vi "Fit VI window to Caller Center.vi"(4 "error in (no error)":errorcluster, 6 "Background VI Ref (Callee's Caller)":refnum<vi>, 7 "VI Ref (calling VI)":refnum<vi>) -> (0 "error out":errorcluster, 3 "VI Ref out":refnum<vi>)   [LabVIEW 2017]
doc: "Resizes and centres the window of VI Ref (calling VI) inside the window of the VI that called it."
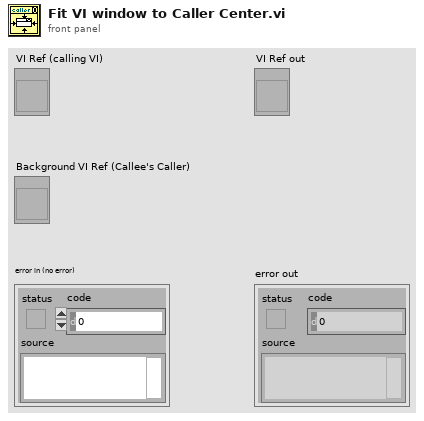
[diagram p1: front panel]
types:
  T1 = typedef "LVRectTypeDef.ctl" = cluster{"Left":i16, "Top":i16, "Right":i16, "Bottom":i16}
  T2 = cluster{"left":i16, "top":i16, "right":i16, "bottom":i16}
  T3 = typedef "LVAllMonitorsDisplayTypeDef.ctl" = cluster{"Bounds":cluster{"Left":i16, "Top":i16, "Right":i16, "Bottom":i16}, "Depth":i16}[]
  T4 = cluster{"Left":i16, "Top":i16, "Right":i16, "Bottom":i16}
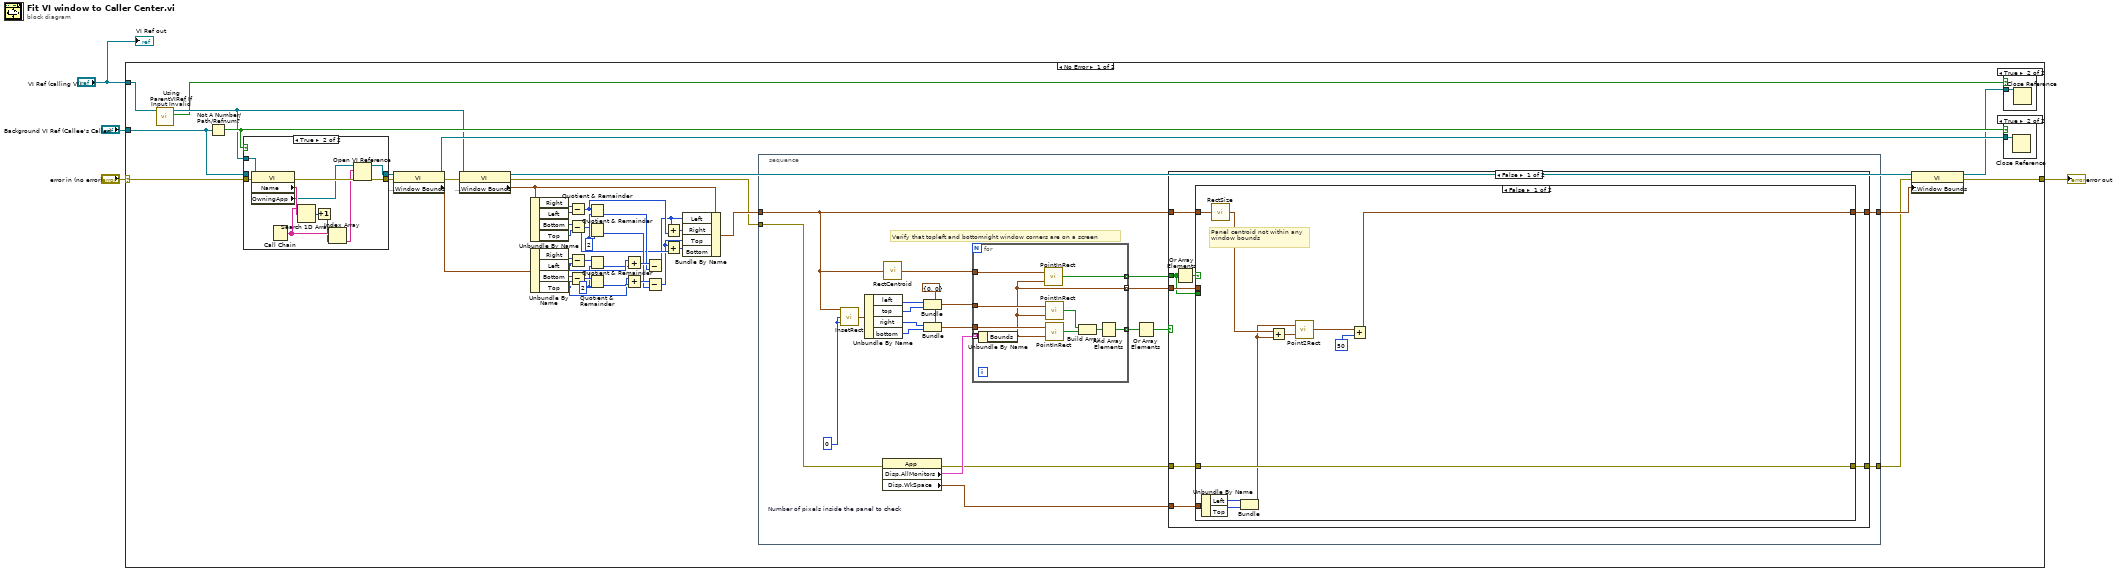
[diagram p0: block diagram]
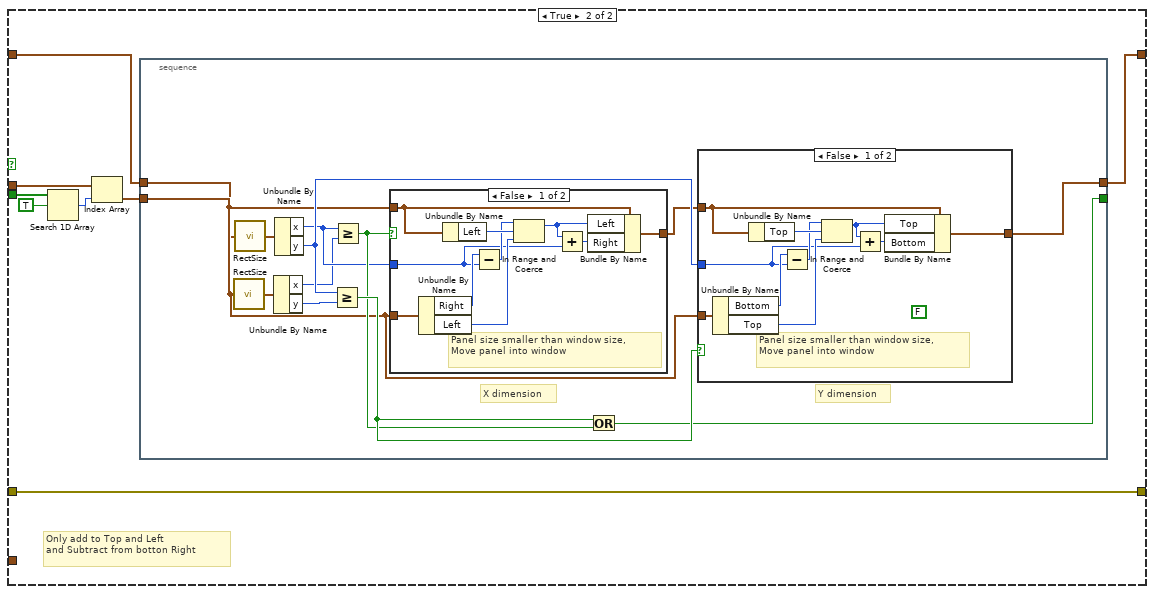
[diagram p2: hidden frame]
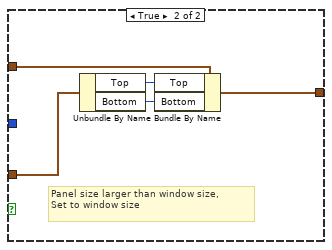
[diagram p3: hidden frame]
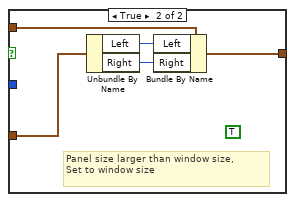
[diagram p4: hidden frame]
diagram:
  n1 = case shown="No Error" "error in (no error)" {
    selector: "error in (no error)" -> [w23 w166]
    tunnel: [w47 w166] -> w4
    tunnel: "Background VI Ref (Callee's Caller)" -> [w19 _]
    tunnel: "VI Ref (calling VI)" -> [w20 _]
    frame No Error {
      w40 = i16 2 ("y")
      w24 = i16 2 ("y")
      n2 = call "Using ParentVIRef If Input Invalid.vi"("VI Ref (calling VI)"=w20) -> ("Using Parent Ref(Need to Destroy)"=w7:bool, "VI Ref"=w15:refnum<vi>)  [unwired: 5 in]
      n3 = Not A Number/Path/Refnum?(number/path/refnum=w19) -> (NaN/Path/Refnum?=w21:bool)
      n4 = case shown="True" w21 {
        tunnel: w19 -> [w154 _]
        tunnel: [w154 w160] -> w18
        tunnel: w15 -> [_ w165]
        tunnel: w23 -> [w153 w164]
        tunnel: [w153 w161] -> w22
        frame False {
        }
        frame True {
          n5 = property class="VI"(reference=w165, error in=w164) -> (error out=w162:errorcluster, "Name"=w163:string, "OwningApp"=w157:refnum<vi>)  [unwired: 1 out]
          n6 = Call Chain() -> (call chain=w159:string[])
          n7 = Search 1D Array(1D array=w159, element=w163) -> (index of element=w156:i32)  [unwired: 1 in]
          n8 = Increment(x=w156) -> (x+1=w155:i32)
          n9 = Index Array(array=w159, index=w155) -> (element=w158:string)
          n10 = Open VI Reference(application reference (local)=w157, vi path=w158, error in (no error)=w162) -> (vi reference=w160:refnum<vi>, error out=w161:errorcluster)  [unwired: 3 in]
        }
      }
      n11 = property class="VI"(reference=w18, error in=w22) -> (reference out=w17:refnum<vi>, error out=w41:errorcluster, "Front Panel Window:Window Bounds"=w46:T1)
      n12 = property class="VI"(reference=w15, error in=w41) -> (reference out=w27:refnum<vi>, error out=w6:errorcluster, "Front Panel Window:Window Bounds"=w10:T1)
      n13 = Unbundle By Name(w10) -> ("Right"=w36:i16, "Left"=w37:i16, "Bottom"=w38:i16, "Top"=w39:i16)
      n14 = Unbundle By Name(w46) -> ("Right"=w45:i16, "Left"=w35:i16, "Bottom"=w44:i16, "Top"=w32:i16)
      n15 = Subtract(x=w36, y=w37) -> (x-y=w26:i16)
      n16 = Subtract(x=w38, y=w39) -> (x-y=w25:i16)
      n17 = Subtract(x=w45, y=w35) -> (x-y=w43:i16)
      n18 = Subtract(x=w44, y=w32) -> (x-y=w42:i16)
      n19 = Quotient & Remainder(x=w26, y=w40) -> (floor(x/y)=w30:i16)  [unwired: 1 out]
      n20 = Quotient & Remainder(x=w25, y=w40) -> (floor(x/y)=w28:i16)  [unwired: 1 out]
      n21 = Quotient & Remainder(x=w43, y=w24) -> (floor(x/y)=w34:i16)  [unwired: 1 out]
      n22 = Quotient & Remainder(x=w42, y=w24) -> (floor(x/y)=w33:i16)  [unwired: 1 out]
      n23 = Add(x=w35, y=w34) -> (x+y=w31:i16)
      n24 = Add(x=w32, y=w33) -> (x+y=w29:i16)
      n25 = Subtract(x=w31, y=w30) -> (x-y=w13:i16)
      n26 = Subtract(x=w29, y=w28) -> (x-y=w12:i16)
      n27 = Add(x=w13, y=w26) -> (x+y=w11:i16)
      n28 = Add(x=w12, y=w25) -> (x+y=w14:i16)
      n29 = Bundle By Name(cluster=w10, "Left"=w13, "Right"=w11, "Top"=w12, "Bottom"=w14) -> (w9:T1)
      n30 = stacked-sequence {
        tunnel: [w58] -> w5
        tunnel: [w49] -> w8
        tunnel: w6 -> [w51]
        tunnel: w9 -> [w65]
        frame #0 {
          w60 = i16 0  # Number of pixels inside the panel to check
          w64 = cluster{"x":i16, "y":i16} {"x"=0, "y"=0} ("point")
          # "Verify that topleft and bottomright window corners are on a screen"
          n31 = call <vilib>:"InsetRect.vi"("dv"=w60, "dh"=w60, "rect"=w65) -> ("inset rect"=w54:T2)
          n32 = Unbundle By Name(w54) -> ("left"=w52:i16, "top"=w53:i16, "right"=w61:i16, "bottom"=w62:i16)
          n33 = property class="App"(error in=w51) -> (error out=w48:errorcluster, "Disp.AllMonitors"=w50:T3, "Disp.WkSpace"=w59:T1)  [unwired: 1 in, 1 out]
          n34 = call <vilib>:"RectCentroid.vi"("rect"=w65) -> ("point"=w66:cluster{"x":i16, "y":i16})
          n35 = Bundle(cluster=w64, "x"=w52, "y"=w53) -> (w55:cluster{"x":i16, "y":i16})
          n36 = Bundle(cluster=w64, "x"=w61, "y"=w62) -> (w63:cluster{"x":i16, "y":i16})
          n37 = for {
            tunnel: w50 -> [w150] mode=indexing
            tunnel: w55 -> [w149]
            tunnel: [w145] -> w56 mode=indexing
            tunnel: w63 -> [w144]
            tunnel: w66 -> [w143]
            tunnel: [w142] -> w67 mode=indexing
            tunnel: [w141] -> w68 mode=indexing
            n38 = Unbundle By Name(w150) -> ("Bounds"=w141:T4)
            n39 = call <vilib>:"PointInRect.vi"("rect"=w141, "point"=w143) -> ("pt in rect"=w142:bool)
            n40 = call <vilib>:"PointInRect.vi"("rect"=w141, "point"=w149) -> ("pt in rect"=w148:bool)
            n41 = call <vilib>:"PointInRect.vi"("rect"=w141, "point"=w144) -> ("pt in rect"=w147:bool)
            n42 = Build Array(w148, w147) -> (w146:bool[])
            n43 = And Array Elements(Boolean array=w146) -> (logical AND=w145:bool)
          }
          n44 = Or Array Elements(Boolean array=w56) -> (logical OR=w57:bool)
          n45 = case shown="False" w57 {
            tunnel: w48 -> [w71 w140]
            tunnel: [w70 w140] -> w58
            tunnel: w65 -> [w75 w139]
            tunnel: [w74 w139] -> w49
            tunnel: w59 -> [w76 _]
            tunnel: w67 -> [w69 _]
            tunnel: w68 -> [w72 _]
            frame False {
              n46 = Or Array Elements(Boolean array=w69) -> (logical OR=w73:bool)
              n47 = case shown="False" w73 {
                tunnel: w76 -> [w87 _]
                tunnel: w75 -> [w83 w90]
                tunnel: [w81 w88] -> w74
                tunnel: w72 -> [_ w92]
                tunnel: w71 -> [w80 w95]
                tunnel: [w80 w95] -> w70
                tunnel: w69 -> [_ w94]
                frame False {
                  # "Panel centroid not within any\nwindow bounds"
                  n48 = Unbundle By Name(w87) -> ("Left"=w86:i16, "Top"=w85:i16)
                  n49 = call <vilib>:"RectSize.vi"("rect"=w83) -> ("point"=w79:cluster{"x":i16, "y":i16})
                  n50 = Bundle("Left"=w86, "Top"=w85) -> (w77:cluster{"Left":i16, "Top":i16})  [unwired: 1 in]
                  n51 = Add(x=w79, y=w77) -> (x+y=w78:cluster{i16, i16})
                  n52 = call <vilib>:"Point2Rect.vi"("point b"=w78, "point a"=w77) -> ("rect"=w82:T2)
                  n53 = Add(x=w82, y=i16 50) -> (x+y=w81:T2)
                }
                frame True {
                  # "Only add to Top and Left\nand Subtract from botton Right"
                  n54 = Search 1D Array(1D array=w94, element=TRUE) -> (index of element=w91:i32)  [unwired: 1 in]
                  n55 = Index Array(array=w92, index=w91) -> (element=w89:T4)
                  n56 = stacked-sequence {
                    tunnel: [w96] -> _
                    tunnel: [w106] -> w88
                    tunnel: w89 -> [w105]
                    tunnel: w90 -> [w97]
                    frame #0 {
                      # "X dimension"
                      # "Y dimension"
                      n57 = call <vilib>:"RectSize.vi"("rect"=w105) -> ("point"=w99:cluster{"x":i16, "y":i16})
                      n58 = call <vilib>:"RectSize.vi"("rect"=w97) -> ("point"=w98:cluster{"x":i16, "y":i16})
                      n59 = Unbundle By Name(w99) -> ("x"=w100:i16, "y"=w103:i16)
                      n60 = Unbundle By Name(w98) -> ("x"=w101:i16, "y"=w104:i16)
                      n61 = Greater Or Equal?(x=w104, y=w103) -> (x >= y?=w108:bool)
                      n62 = Greater Or Equal?(x=w101, y=w100) -> (x >= y?=w107:bool)
                      n63 = case shown="False" w107 {
                        tunnel: w105 -> [w133 w134]
                        tunnel: w97 -> [w125 w135]
                        tunnel: w101 -> [w126 _]
                        tunnel: [w124 w136] -> w102
                        frame False {
                          # "Panel size smaller than window size,\nMove panel into window"
                          n64 = Unbundle By Name(w133) -> ("Right"=w129:i16, "Left"=w131:i16)
                          n65 = Unbundle By Name(w125) -> ("Left"=w132:i16)
                          n66 = Subtract(x=w129, y=w126) -> (x-y=w130:i16)
                          n67 = In Range and Coerce(upper limit=w130, x=w132, lower limit=w131) -> (coerced(x)=w128:i16)  [unwired: 1 out]
                          n68 = Add(x=w128, y=w126) -> (x+y=w127:i16)
                          n69 = Bundle By Name(cluster=w125, "Left"=w128, "Right"=w127) -> (w124:T1)
                        }
                        frame True {
                          (unwired) TRUE
                          # "Panel size larger than window size,\nSet to window size"
                          n70 = Unbundle By Name(w134) -> ("Left"=w138:i16, "Right"=w137:i16)
                          n71 = Bundle By Name(cluster=w135, "Left"=w138, "Right"=w137) -> (w136:T1)
                        }
                      }
                      n72 = Or(x=w108, y=w107) -> (x .or. y?=w96:bool)
                      n73 = case shown="False" w108 {
                        tunnel: w105 -> [w118 w123]
                        tunnel: w102 -> [w110 w119]
                        tunnel: w104 -> [w111 _]
                        tunnel: [w109 w120] -> w106
                        frame False {
                          (unwired) FALSE
                          # "Panel size smaller than window size,\nMove panel into window"
                          n74 = Unbundle By Name(w118) -> ("Bottom"=w114:i16, "Top"=w116:i16)
                          n75 = Unbundle By Name(w110) -> ("Top"=w117:i16)
                          n76 = Subtract(x=w114, y=w111) -> (x-y=w115:i16)
                          n77 = In Range and Coerce(upper limit=w115, x=w117, lower limit=w116) -> (coerced(x)=w113:i16)  [unwired: 1 out]
                          n78 = Add(x=w113, y=w111) -> (x+y=w112:i16)
                          n79 = Bundle By Name(cluster=w110, "Top"=w113, "Bottom"=w112) -> (w109:T1)
                        }
                        frame True {
                          # "Panel size larger than window size,\nSet to window size"
                          n80 = Unbundle By Name(w123) -> ("Top"=w122:i16, "Bottom"=w121:i16)
                          n81 = Bundle By Name(cluster=w119, "Top"=w122, "Bottom"=w121) -> (w120:T1)
                        }
                      }
                    }
                  }
                }
              }
            }
            frame True {
            }
          }
        }
      }
      n82 = property class="VI"(reference=w27, error in=w5, "Front Panel Window:Window Bounds"=w8) -> (reference out=w16:refnum<vi>, error out=w47:errorcluster)
      n83 = case shown="True" w21 {
        tunnel: w17 -> [_ w152]
        frame False {
        }
        frame True {
          n84 = Close Reference(reference=w152) -> ()  [unwired: 1 in, 1 out]
        }
      }
      n85 = case shown="True" w7 {
        tunnel: w16 -> [_ w151]
        frame False {
        }
        frame True {
          n86 = Close Reference(reference=w151) -> ()  [unwired: 1 in, 1 out]
        }
      }
    }
    frame Error {
    }
  }
  "error out" <- w4
  "VI Ref out" <- "VI Ref (calling VI)"
